vi "Open Front Panel(Event Callback).vi"(4 "user event":refnum<user-event>, 5 "Event Data":cluster{"sender":refnum<k24>, "e":refnum<k24>}, 6 "Control Ref":refnum<k24>, 7 "Event Common Data":T1) -> ()   [LabVIEW 2019, in "Test Bench Tools.lvlib"]
uses:
  Test Bench Tools.lvlib
  System.Windows.Forms
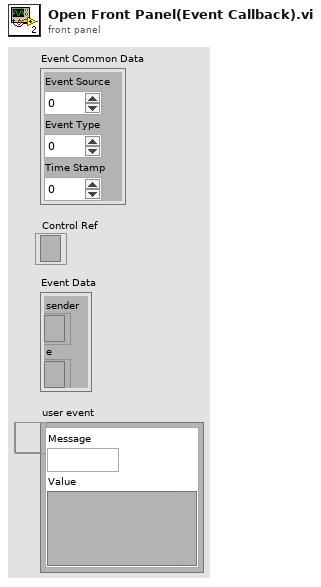
[diagram p1: front panel]
types:
  T1 = cluster{"Event Source":i32, "Event Type":u32, "Time Stamp":u32}
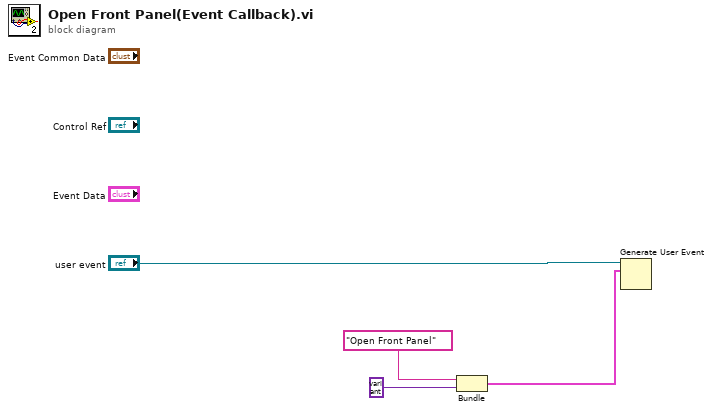
[diagram p0: block diagram]
diagram:
  n1 = Bundle("event data"="Open Front Panel", variant) -> (w2:cluster{"event data":string, variant})  [unwired: 1 in]
  n2 = Generate User Event(user event="user event", event data cluster=w2) -> ()  [unwired: 2 in, 2 out]
